vi "Register for Broadcast Events.vi"(8 "error in (no error)":errorcluster, 10 "Event Registration Refnum In":refnum<event-registration>, 11 "Process In":refnum<class "Debug View.lvclass">) -> (0 "error out":errorcluster, 2 "Event Registration Refnum Out":refnum<event-registration>, 3 "Process Out":refnum<class "Debug View.lvclass">)   [LabVIEW 2020, in "Debug View.lvclass"]
doc: "Returns a registration to broadcase messages from the process and any owned processes."
uses:
  Debug View.lvclass
  Protected/Broadcasting/Broadcast Message Cluster.ctl
  Debug View.lvclass/Debug View.ctl
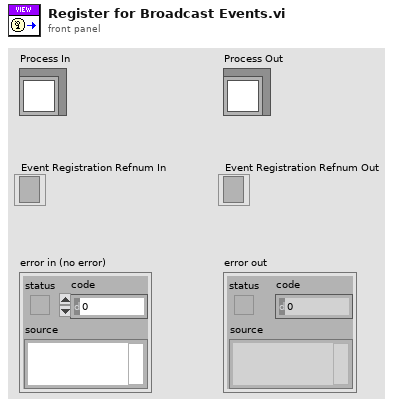
[diagram p1: front panel]
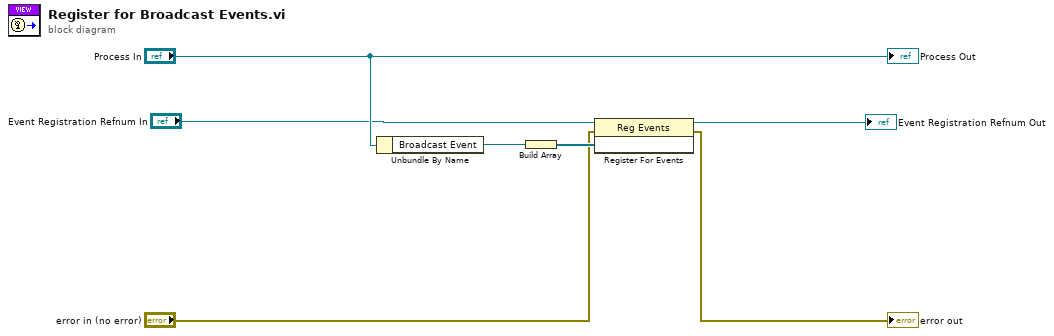
[diagram p0: block diagram]
diagram:
  n1 = Unbundle By Name("Process In") -> ("Broadcast Event"=w6:refnum<user-event>)
  n2 = Build Array(w6) -> (w3:refnum<user-event>[])
  n3 = register-events(reference="Event Registration Refnum In", error in="error in (no error)", w3) -> (reference out=→"Event Registration Refnum Out":refnum<event-registration>, error out=→"error out":errorcluster)
  "Process Out" <- "Process In"
